vi "Get RB Color Channels.vi"(8 "Error In":errorcluster, 10 "Image In":T1(plugin-control)) -> (0 "Error Out":errorcluster, 2 "Blue Channel":T1(plugin-control), 3 "Red Channel":T1(plugin-control))   [LabVIEW 2018]
uses:
  <vilib>/vision/NI_Vision_Development_Module.lvlib
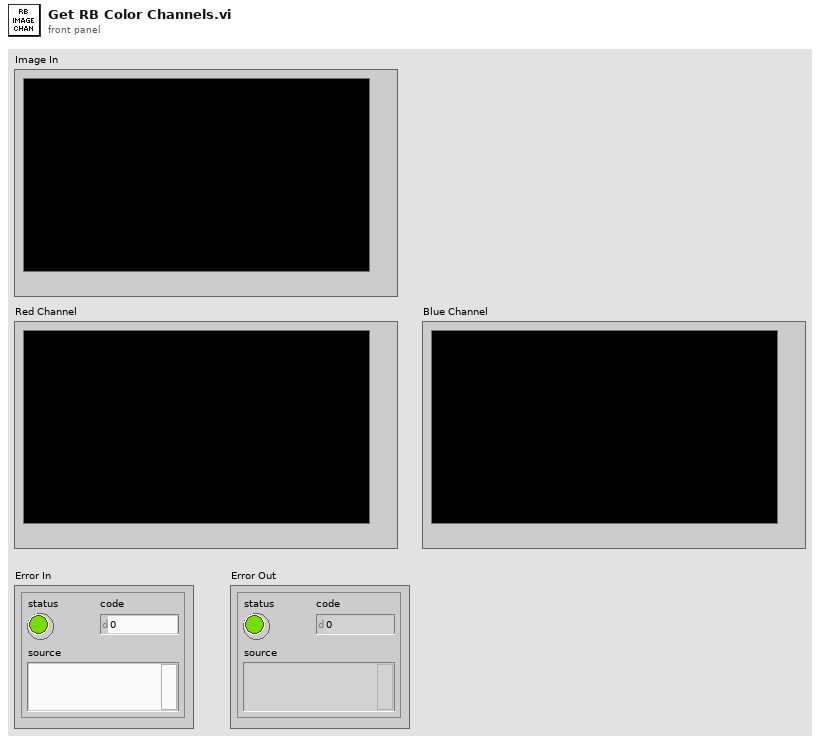
[diagram p1: front panel]
types:
  T1 = typedef "IMAQ Image.ctl" = refnum<image>
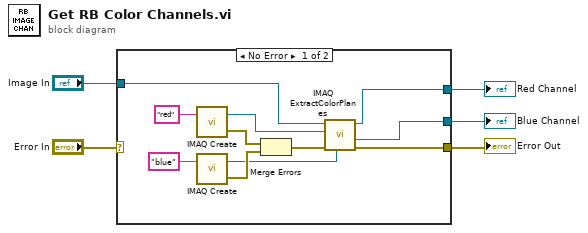
[diagram p0: block diagram]
diagram:
  n1 = case shown="No Error" "Error In" {
    selector: "Error In" -> [_ w17]
    tunnel: "Image In" -> [w10 _]
    tunnel: [w11 w17] -> w3
    tunnel: [w7 _] -> w2
    tunnel: [w6 _] -> w1
    frame No Error {
      n2 = call "IMAQ Create"("Image Name"="red") -> ("New Image"=w9:T1, "error out"=w14:errorcluster)  [unwired: 4 in]
      n3 = call "IMAQ Create"("Image Name"="blue") -> ("New Image"=w8:T1, "error out"=w13:errorcluster)  [unwired: 4 in]
      n4 = Merge Errors(w14, w13) -> (w12:errorcluster)
      n5 = call "IMAQ ExtractColorPlanes"("Blue or Luma or Val or Inten Plane"=w8, "error in (no error)"=w12, "Red or Hue Plane"=w9, "Image Src"=w10) -> ("error out"=w11:errorcluster, "Blue or Luma or Val or Inten Plane out"=w6:T1, "Red or Hue Plane out"=w7:T1)  [unwired: 4 in, 1 out]
    }
    frame Error {
    }
  }
  "Error Out" <- w3
  "Red Channel" <- w2
  "Blue Channel" <- w1
